vi "onDisconnection.vi"(8 "error in (no error)":errorcluster, 11 "WSConnection in":refnum<class "WebsocketsConnection.lvclass">) -> (0 "error out":errorcluster, 3 "No Connection":refnum<class "WebsocketsConnection.lvclass">)   [LabVIEW 2013, in "MQTT_Websockets.lvlib" / "WebsocketsConnection.lvclass"]
uses:
  WebsocketsConnection.lvclass
  <vilib>/LabVIEW Open Source Project/MQTT Connection/MQTT_Connection/Connection/Connection.lvclass
  WebsocketsConnection.lvclass/WebsocketsConnection.ctl
  <vilib>/MediaMongrels Ltd/WebSockets/WebSockets/WebSocket/WebSocket.lvclass
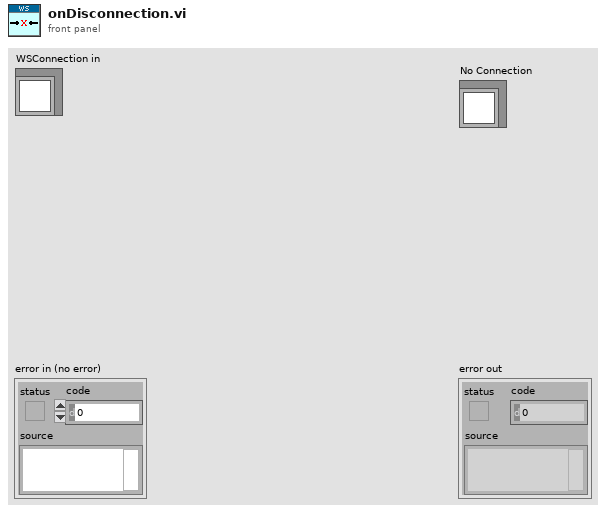
[diagram p1: front panel]
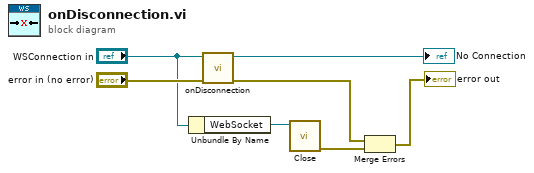
[diagram p0: block diagram]
diagram:
  n1 = Unbundle By Name("WSConnection in") -> ("WebSocket"=w2:refnum<class "WebSocket.lvclass">)
  n2 = call-parent "onDisconnection.vi"("error in (no error)"="error in (no error)", "Connection"="WSConnection in") -> ("error out"=w5:errorcluster, "No connection"=→"No Connection":refnum<class "WebsocketsConnection.lvclass">)  [unwired: 8 in]
  n3 = call-dynamic "Close.vi"("WebSocket in"=w2) -> ("error out"=w1:errorcluster)  [unwired: 10 in]
  n4 = Merge Errors(w5, w1) -> (→"error out":errorcluster)
